vi "AI RAG Initialize.vi"(0 "Python RAG Script":path, 1 "ProcessMdFuncName":string, 2 "RetrContextFuncName":string, 5 "Knowledge Base Name":string, 7 "Chroma Database Folder":path, 11 "error in (no error)":errorcluster, 12 "Embedding Model URL":string, 13 "Embedding Model Name":string) -> (15 "error out":errorcluster)   [LabVIEW 2023, in "LabVIEW RAG.lvlib"]
uses:
  LabVIEW RAG.lvlib
  AI RAG Globals.vi
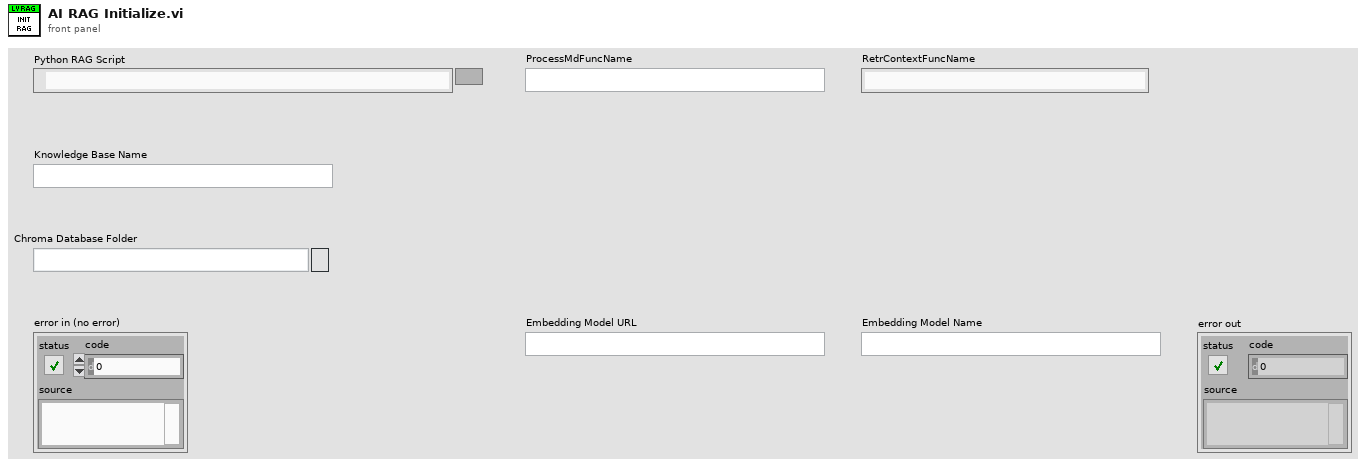
[diagram p1: front panel]
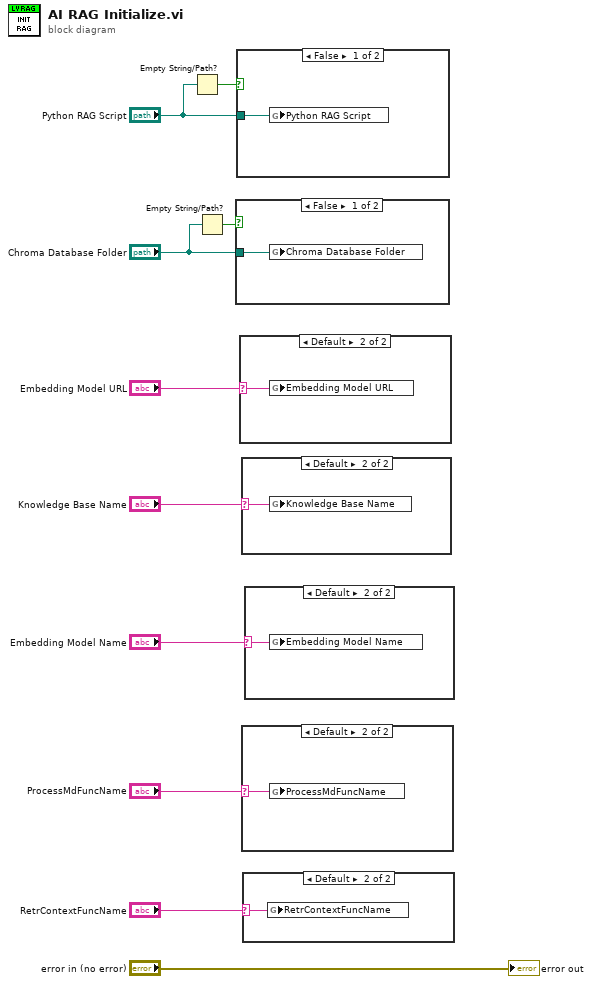
[diagram p0: block diagram]
diagram:
  n1 = Empty String/Path?(string/path="Python RAG Script") -> (empty?=w4:bool)
  n2 = Empty String/Path?(string/path="Chroma Database Folder") -> (empty?=w2:bool)
  n3 = case shown="False" w2 {
    tunnel: "Chroma Database Folder" -> [w11 _]
    frame False {
      n4 = global write "AI RAG Globals.vi" "Chroma Database Folder"(w11) -> ()
    }
    frame True {
    }
  }
  n5 = case shown="False" w4 {
    tunnel: "Python RAG Script" -> [w12 _]
    frame False {
      n6 = global write "AI RAG Globals.vi" "Python RAG Script"(w12) -> ()
    }
    frame True {
    }
  }
  n7 = case shown="Default" "Embedding Model URL" {
    selector: "Embedding Model URL" -> [_ w13]
    frame "" {
    }
    frame Default {
      n8 = global write "AI RAG Globals.vi" "Embedding Model URL"(w13) -> ()
    }
  }
  n9 = case shown="Default" "Knowledge Base Name" {
    selector: "Knowledge Base Name" -> [_ w14]
    frame "" {
    }
    frame Default {
      n10 = global write "AI RAG Globals.vi" "Knowledge Base Name"(w14) -> ()
    }
  }
  n11 = case shown="Default" "ProcessMdFuncName" {
    selector: "ProcessMdFuncName" -> [_ w15]
    frame "" {
    }
    frame Default {
      n12 = global write "AI RAG Globals.vi" "ProcessMdFuncName"(w15) -> ()
    }
  }
  n13 = case shown="Default" "RetrContextFuncName" {
    selector: "RetrContextFuncName" -> [_ w16]
    frame "" {
    }
    frame Default {
      n14 = global write "AI RAG Globals.vi" "RetrContextFuncName"(w16) -> ()
    }
  }
  n15 = case shown="Default" "Embedding Model Name" {
    selector: "Embedding Model Name" -> [_ w17]
    frame "" {
    }
    frame Default {
      n16 = global write "AI RAG Globals.vi" "Embedding Model Name"(w17) -> ()
    }
  }
  "error out" <- "error in (no error)"
